vi "blinking a led.vi"() -> ()   [LabVIEW 2019]
uses:
  <vilib>/LabVIEW Interface for Arduino/Type Defs/Connection Type.ctl
  <vilib>/LabVIEW Interface for Arduino/Type Defs/Board Type.ctl
  <vilib>/LabVIEW Interface for Arduino/Type Defs/Pin Mode.ctl
  <vilib>/LabVIEW Interface for Arduino/LabVIEW Interface for Arduino.lvlib
panel:
  in  "stop":bool
  in  "VISA resource":refnum<visa-resource-name>
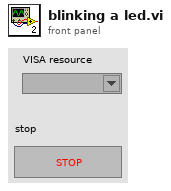
[diagram p1: front panel]
types:
  T1 = typedef "LabVIEW Interface for Arduino.lvlib/Pin Mode.ctl" = enum8{"Input", "Output"}
  T2 = typedef "LabVIEW Interface for Arduino.lvlib/Board Type.ctl" = enum16{"Uno", "Dimuelanove w/Atmega 328", "Mega 2560"}
  T3 = typedef "LabVIEW Interface for Arduino.lvlib/Connection Type.ctl" = enum8{"USB / Serial", "XBEE", "BlueSmirf (Bluetooth)"}
  T4 = typedef "LabVIEW Interface for Arduino.lvlib/Arduino Resource.ctl" = cluster{"VISA resource":refnum<visa-resource-name>, "Board Type":T2, "Connection Type":enum8{"USB / Serial"}, "Bytes Per Packet (15)":u8}
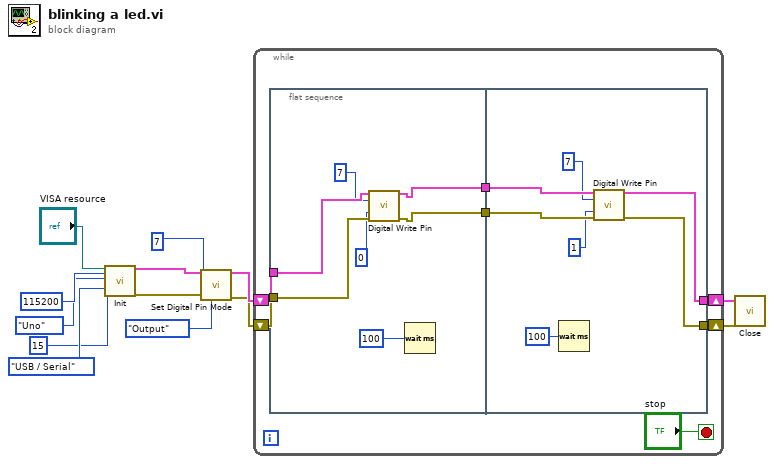
[diagram p0: block diagram]
diagram:
  n1 = call <vilib>:"Init.vi"("VISA resource"="VISA resource", "Baud Rate (115200)"=u32 115200, "Board Type (Uno)"=Board_Type."Uno", "Bytes Per Packet (15)"=u32 15, "Connection Type (USB/Serial)"=Connection_Type."USB / Serial") -> ("Arduino Resource"=w8:T4, "error out"=w7:errorcluster)  [unwired: 13 in]
  n2 = call <vilib>:"Set Digital Pin Mode.vi"("Arduino Resource"=w8, "Digital I/O Pin"=u8 7, "Pin Mode (Input)"=Pin_Mode."Output", "error in"=w7) -> ("Arduino Resource"=w4:T4, "error out"=w3:errorcluster)  [unwired: 10 in]
  n3 = while {
    shift-right: [w16] -> w2
    shift-left: w4 -> [w18]
    shift-right: [w15] -> w1
    shift-left: w3 -> [w17]
    stop <- "stop" stop-if-true
    n4 = flat-sequence {
      tunnel: w18 -> [w27]
      tunnel: w17 -> [w26]
      tunnel: [w22] -> w20
      tunnel: [w23] -> w19
      tunnel: w20 -> [w34]
      tunnel: w19 -> [w33]
      tunnel: [w30] -> w16
      tunnel: [w29] -> w15
      frame #0 {
        n5 = call <vilib>:"Digital Write Pin.vi"("Arduino Resource"=w27, "Digital I/O Pin (0)"=u8 7, "Value (0)"=u8 0, "error in"=w26) -> ("Arduino Resource"=w22:T4, "error out"=w23:errorcluster)  [unwired: 10 in]
        n6 = Wait (ms)(milliseconds to wait=u32 100 ("millisecond timer value")) -> ()  [unwired: 1 out]
      }
      frame #1 {
        n7 = Wait (ms)(milliseconds to wait=u32 100) -> ()  [unwired: 1 out]
        n8 = call <vilib>:"Digital Write Pin.vi"("Arduino Resource"=w34, "Digital I/O Pin (0)"=u8 7, "Value (0)"=u8 1, "error in"=w33) -> ("Arduino Resource"=w30:T4, "error out"=w29:errorcluster)  [unwired: 10 in]
      }
    }
  }
  n9 = call <vilib>:"Close.vi"("Arduino Resource"=w2, "error in"=w1) -> ()  [unwired: 13 in, 1 out]
